vi "BC-Put-Ball_Api.vi"(5 "加速度":dbl=200.0 format="%#_13g", 7 "最高速":dbl=300.0 format="%#_13g", 8 "Error In":errorcluster) -> (0 "Error Out":errorcluster)   [LabVIEW 2019]
uses:
  <vilib>/Platform/TimedLoop/XDataNode/timing_clust.ctl
  <vilib>/Platform/TimedLoop/XDataNode/nitl_modes.ctl
  <vilib>/Platform/TimedLoop/XDataNode/wakeup.ctl
  <vilib>/platform/TimedLoop/XDataNode/XDataNode.xnode
  <vilib>/Platform/TimedLoop/XDataNode/XDNodeRunTimeDep.lvlib
panel:
  in  "Stop":bool
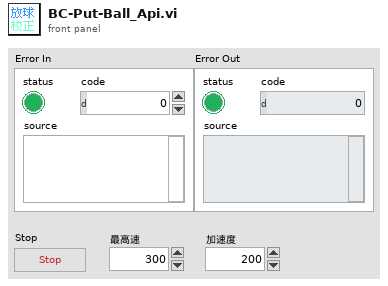
[diagram p1: front panel]
types:
  T1 = typedef "XDNodeRunTimeDep.lvlib/timing_clust.ctl" = cluster{"Expected End [f-1]":u64, "Actual End [f-1]":u64, "Finished Late? [f-1]":bool, "Expected End [i-1]":u64, "Actual End [i-1]":u64, "Finished Late? [i-1]":bool, "Expected Start [i]":u64, "Actual Start [i]":u64, "Expected Start [f]":u64, "Actual Start [f]":u64, "Source Name":string, "Structure Name":string, "Period":i64, "Deadline":i64, "Offset":i64, "Start":i64, "Priority":i32, "Timeout":i32, "Mode":T2, "Wakeup Reason":T3, "Error":errorcluster, "Source Type":string, "Secondary Source Type":string, "Global End Time":u64, "Global Start Time":u64, "Frame Duration":u64, "Iteration Duration":u64, "Assigned CPU":i32, "I/O Scan Engine Mode":u32}
  T2 = typedef "XDNodeRunTimeDep.lvlib/nitl_modes.ctl" = enum32{"No Change", "Process missed periods, maintain original phase", "Discard missed periods, maintain original phase", "Process missed periods, ignore original phase", "Discard missed periods, ignore original phase"}
  T3 = typedef "XDNodeRunTimeDep.lvlib/wakeup.ctl" = enum32{"Normal", "Aborted", "Asynchronous wakeup", "Timing source error", "Timed loop error", "Timeout"}
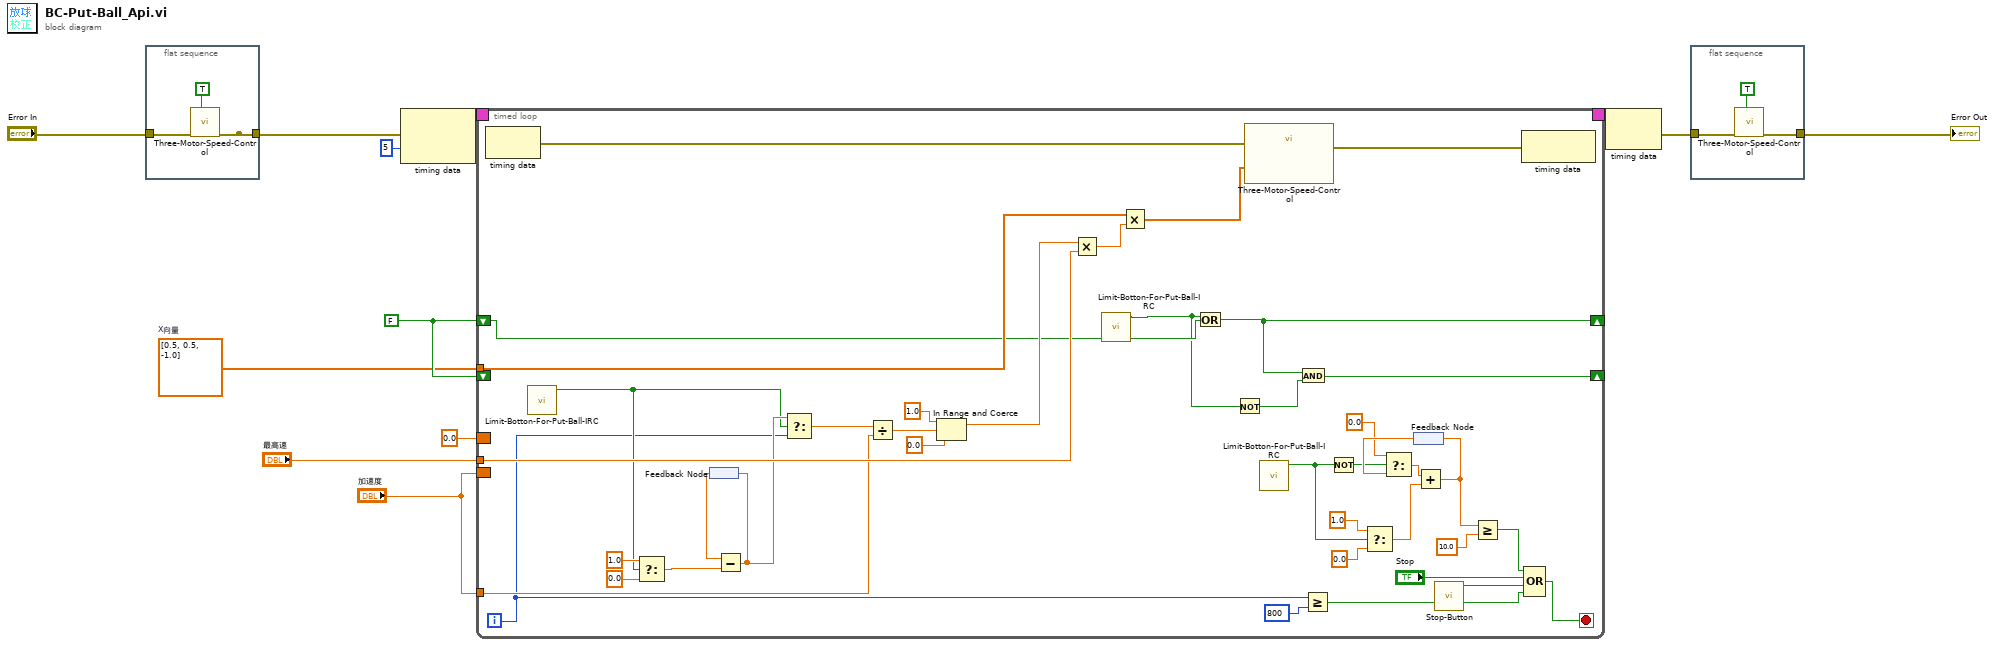
[diagram p0: block diagram]
diagram:
  w6 = dbl[] [0.5, 0.5, -1.0]  # X向量
  w8 = FALSE
  n1 = flat-sequence {
    tunnel: "Error In" -> [w14]
    tunnel: [w13] -> _
    tunnel: [w13] -> w4
    frame #0 {
      n2 = call "Three-Motor-Speed-Control.vi"("Reset"=TRUE, "Error In"=w14) -> ("Error Out"=w13:errorcluster)  [unwired: 9 in]
    }
  }
  n3 = node-c288(w4, i64 5 ("Period")) -> (w12:T1)
  n4 = timed-loop {
    timing: w12 -> [_]
    timing-out: [_] -> w11
    tunnel: "最高速" -> [w50]
    border: "加速度" -> [_]
    tunnel: "加速度" -> [w43]
    tunnel: w6 -> [w36]
    shift-right: [w33] -> _
    shift-left: w8 -> [w32]
    shift-right: [w41] -> _
    shift-left: w8 -> [_]
    border: 0.0 -> [_]
    i -> [w18]
    stop <- w53 stop-if-true
    n5 = node-c288() -> (w55:errorcluster)  [unwired: 1 in]
    n6 = call "Limit-Botton-For-Put-Ball-IRC.vi"() -> ("放球校正微動觸發?"=w30:bool)  [unwired: 10 in, 1 out]
    n7 = Select(t=1.0, s=w30, f=0.0) -> (s? t:f=w48:dbl)
    n8 = feedback #1() -> (w47:dbl)
    n9 = Subtract(x=w47, y=w48) -> (x-y=w46:dbl)
    n10 = feedback-in #1(w46) -> ()
    n11 = Select(t=w46, s=w30, f=w18) -> (s? t:f=w45:dbl)
    n12 = Divide(x=w45, y=w43) -> (x/y=w40:dbl)
    n13 = In Range and Coerce(upper limit=1.0, x=w40, lower limit=0.0) -> (coerced(x)=w37:dbl)  [unwired: 1 out]
    n14 = Multiply(x=w37, y=w50) -> (x*y=w35:dbl)
    n15 = call "Limit-Botton-For-Put-Ball-IRC.vi"() -> ("放球校正微動觸發?"=w31:bool)  [unwired: 10 in, 1 out]
    n16 = Multiply(x=w36, y=w35) -> (x*y=w34:dbl[])
    n17 = Or(x=w31, y=w32) -> (x .or. y?=w33:bool)
    n18 = Not(x=w31) -> (.not. x?=w42:bool)
    n19 = call "Three-Motor-Speed-Control.vi"("Error In"=w55, "速度(秒/度)"=w34) -> ("Error Out"=w54:errorcluster)  [unwired: 9 in]
    n20 = call "Limit-Botton-For-Put-Ball-IRC.vi"() -> ("放球校正微動觸發?"=w19:bool)  [unwired: 10 in, 1 out]
    n21 = And(x=w33, y=w42) -> (x .and. y?=w41:bool)
    n22 = Greater Or Equal?(x=w18, y=800) -> (x >= y?=w16:bool)
    n23 = Not(x=w19) -> (.not. x?=w25:bool)
    n24 = Select(t=1.0, s=w19, f=0.0) -> (s? t:f=w27:dbl)
    n25 = feedback #2() -> (w26:dbl)
    n26 = Select(t=0.0, s=w25, f=w26) -> (s? t:f=w23:dbl)
    n27 = Add(x=w23, y=w27) -> (x+y=w22:dbl)
    n28 = feedback-in #2(w22) -> ()
    n29 = call "Stop-Button.vi"() -> ("顯示按下?"=w51:bool)  [unwired: 10 in, 1 out]
    n30 = Greater Or Equal?(x=w22, y=10.0) -> (x >= y?=w20:bool)
    n31 = node-c288(w54) -> ()  [unwired: 1 out]
    n32 = Compound Arithmetic op=OR(w20, "Stop", w51, w16) -> (w53:bool)
  }
  n33 = node-c288(w11) -> (w7:errorcluster)
  n34 = flat-sequence {
    tunnel: w7 -> [w62]
    tunnel: [w61] -> w3
    frame #0 {
      n35 = call "Three-Motor-Speed-Control.vi"("Reset"=TRUE, "Error In"=w62) -> ("Error Out"=w61:errorcluster)  [unwired: 9 in]
    }
  }
  "Error Out" <- w3
